vi "ExecuteCommand.vi"(10 "Params":string[][](array[string]), 11 "Command":string) -> ()   [LabVIEW 2017]
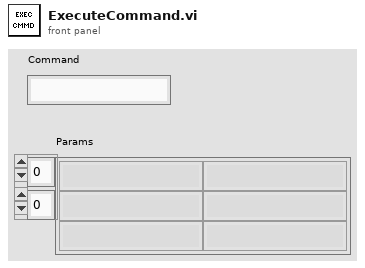
[diagram p1: front panel]
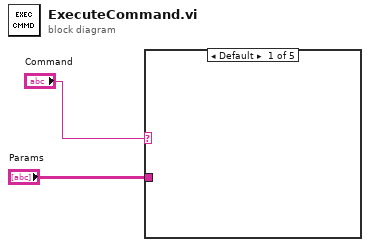
[diagram p0: block diagram]
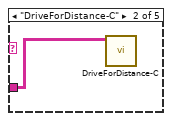
[diagram p2: hidden frame]
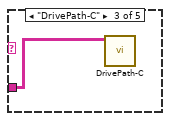
[diagram p3: hidden frame]
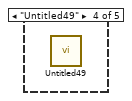
[diagram p4: hidden frame]
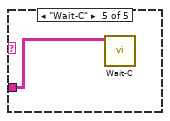
[diagram p5: hidden frame]
diagram:
  n1 = case shown="Default" "Command" {
    tunnel: "Params" -> [_ w3 w4 _ w5]
    frame Default {
    }
    frame "DriveForDistance-C" {
      n2 = call "DriveForDistance-C.vi"("Params"=w3) -> ()  [unwired: 11 in]
    }
    frame "DrivePath-C" {
      n3 = call "DrivePath-C.vi"("Params"=w4) -> ()  [unwired: 11 in]
    }
    frame "Untitled49" {
      n4 = call "Untitled49.vi"() -> ()  [unwired: 12 in]
    }
    frame "Wait-C" {
      n5 = call "Wait-C.vi"("Params"=w5) -> ()  [unwired: 11 in]
    }
  }
